vi "ACT_STOP.vi"(8 "error in (no error)":errorcluster, 11 "NeedleValve in":refnum<class "NeedleValve.lvclass">) -> (0 "error out":errorcluster, 3 "NeedleValve out":refnum<class "NeedleValve.lvclass">)   [LabVIEW 2019, in "NeedleValve.lvclass"]
uses:
  NeedleValve.lvclass
  NeedleValve.lvclass/NeedleValve.ctl
  modbus engine custom/MB_ENGINE_class/cmd enum.ctl
  modbus engine custom/MB_ENGINE_class/MB_ENGINE.lvclass
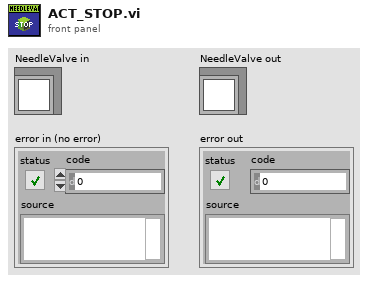
[diagram p1: front panel]
types:
  T1 = typedef "MB_ENGINE.lvclass/cmd enum.ctl" = u16
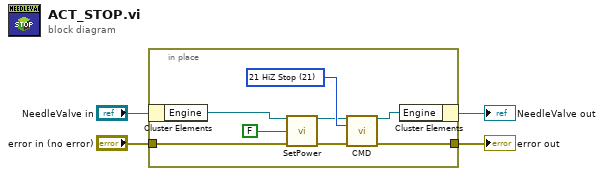
[diagram p0: block diagram]
diagram:
  n1 = in-place {
    in-place-border: "error in (no error)" -> [w6]
    in-place-border: [w5] -> w4
    w12 = T1 21 items=["0 Idle"=0, "1 GoTo Absolute Position"=1, "2 GoTo Relative"=2, "10 GoTo Home Position"=10, "11 Set Home Position"=11, "12 Set FindHome Mode"=12, "13 Reset FindHome Mode"=13, "14 Get FindHome State"=14, "20 Hard Stop"=20, "21 HiZ Stop"=21, "22 Soft Stop"=22, "30 Clear Fault"=30, "40 Encoder Set Home"=40, "70 Driver Init"=70] ("cmd to write")
    n2 = in-place-cluster #1("NeedleValve in") -> ("Engine"=w8:refnum<class "MB_ENGINE.lvclass">)
    n3 = call "SetPower.vi"("class data in"=w8, "On"=FALSE, "error in (no error)"=w6) -> ("class data out"=w9:refnum<class "MB_ENGINE.lvclass">, "error out"=w10:errorcluster)  [unwired: 11 in]
    n4 = call "CMD.vi"("class data in"=w9, "cmd to write"=w12, "error in (no error)"=w10) -> ("class data out"=w7:refnum<class "MB_ENGINE.lvclass">, "error out"=w5:errorcluster)  [unwired: 11 in]
    n5 = in-place-cluster #1("Engine"=w7) -> (→"NeedleValve out":refnum<class "NeedleValve.lvclass">)
  }
  "error out" <- w4
